vi "VCL_2_TSV.vi"(8 "error in (no error)":errorcluster, 11 "Path to VCL file":path) -> (0 "error out":errorcluster, 1 "standard output":string, 2 "path to VCL file":path, 3 "path to logfile directory":path)   [LabVIEW 2016, in "VCL_2_DSC.lvclass"]
uses:
  VCL_2_DSC.lvclass
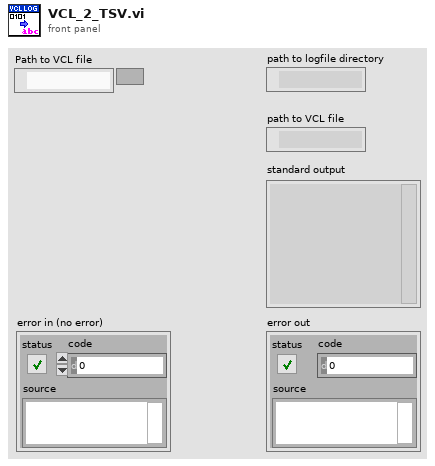
[diagram p1: front panel]
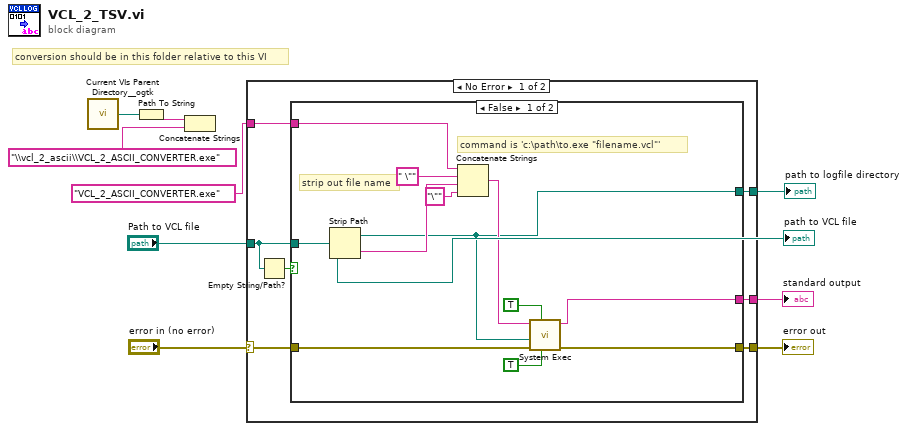
[diagram p0: block diagram]
diagram:
  # "conversion should be in this folder relative to this VI"
  n1 = call <userlib>:"Current VIs Parent Directory__ogtk.vi"() -> ("Parent Directory (+ Relative)"=w6:path)  [unwired: 5 in]
  n2 = Path To String(path=w6) -> (string=w5:string)
  n3 = Concatenate Strings(w5, "\\vcl_2_ascii\\VCL_2_ASCII_CONVERTER.exe" ("full path to VCL_2_ASCII_CONVERTER.exe")) -> ()  [unwired: 1 out]
  n4 = case shown="No Error" "error in (no error)" {
    selector: "error in (no error)" -> [w10 w30]
    tunnel: [w16 w30] -> w9
    tunnel: [w15 _] -> w8
    tunnel: [w14 _] -> w7
    tunnel: "VCL_2_ASCII_CONVERTER.exe" ("full path to VCL_2_ASCII_CONVERTER.exe") -> [w13 _]
    tunnel: "Path to VCL file" -> [w11 _]
    frame No Error {
      n5 = Empty String/Path?(string/path=w11) -> (empty?=w12:bool)
      n6 = case shown="False" w12 {
        tunnel: w10 -> [w28 w29]
        tunnel: [w27 w29] -> w16
        tunnel: [w22 _] -> w15
        tunnel: [w17 _] -> w14
        tunnel: w11 -> [w21 _]
        tunnel: w13 -> [w20 _]
        frame False {
          # "command is 'c:\\path\\to.exe \"filename.vcl\"'"
          # "strip out file name"
          n7 = Strip Path(path=w21) -> (stripped path=w17:path, name=w24:string)
          n8 = Concatenate Strings(w20, " \"" ("string"), w24, "\"" ("string")) -> (w25:string)
          n9 = call <vilib>:"System Exec.vi"("run minimized? (F)"=TRUE, "wait until completion? (T)"=TRUE, "error in (no error)"=w28, "working directory"=w17, "command line"=w25) -> ("error out"=w27:errorcluster, "standard output"=w22:string)  [unwired: 3 in, 2 out]
        }
        frame True {
        }
      }
    }
    frame Error {
    }
  }
  "standard output" <- w8
  "error out" <- w9
  "path to logfile directory" <- w7
  "path to VCL file" <- "Path to VCL file"
